vi "loop-time-sample-rate-calc-check.vi"(8 "sample-rate-Hz":dbl=4.0, 11 "millisecond timer value in":u32) -> (0 "Loop Hz":dbl format="%-#3.3f", 1 "Loop Time (mS)":u32, 2 "sample-rate-delay-mS":u32, 3 "millisecond timer value out":u32)   [LabVIEW 2024]
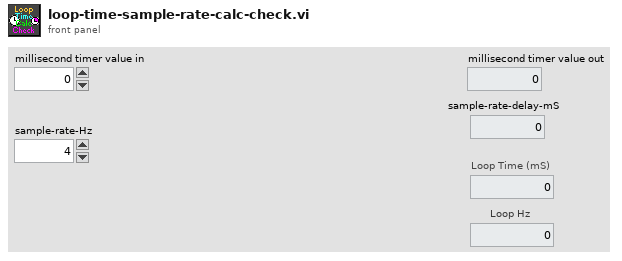
[diagram p1: front panel]
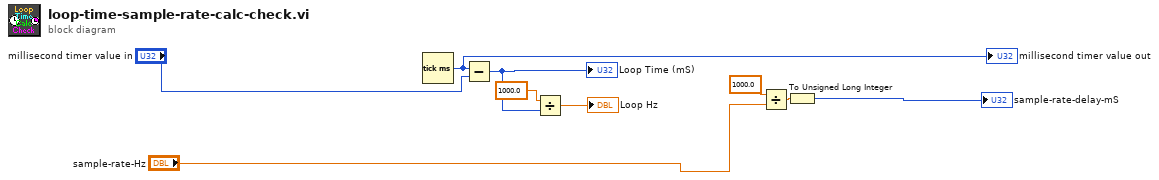
[diagram p0: block diagram]
diagram:
  n1 = Tick Count (ms)() -> (millisecond timer value=w5:u32)
  "millisecond timer value out" <- w5
  n2 = Subtract(x=w5, y="millisecond timer value in") -> (x-y=w8:u32)
  "Loop Time (mS)" <- w8
  n3 = Divide(x=1000.0 ("milliseconds to wait"), y=w8) -> (x/y=→"Loop Hz":dbl)
  n4 = Divide(x=1000.0 ("milliseconds to wait"), y="sample-rate-Hz") -> (x/y=w3:dbl)
  n5 = To Unsigned Long Integer(number=w3) -> (unsigned 32bit integer=→"sample-rate-delay-mS":u32)
